vi "powermeter-main.vi"(3 "Perform Powermeter Auto Zero?":bool, 4 "error in (no error)":errorcluster, 5 "input-wavelength":i32, 6 "Set Wavelength?":bool, 7 "VISA in":refnum<visa-resource-name>="COM1") -> (0 "error out":errorcluster, 1 "output-wavelength":i32, 2 "power (µW)":dbl)   [LabVIEW 2015]
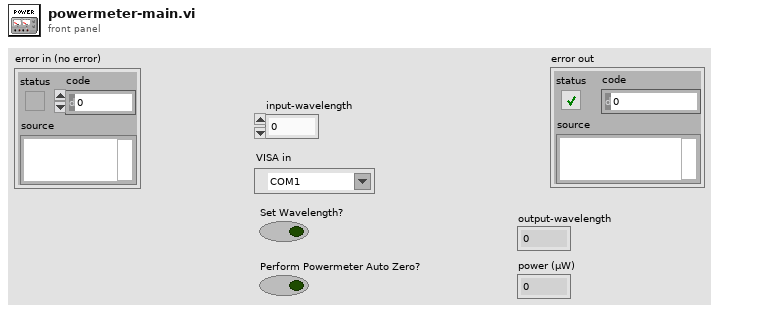
[diagram p1: front panel]
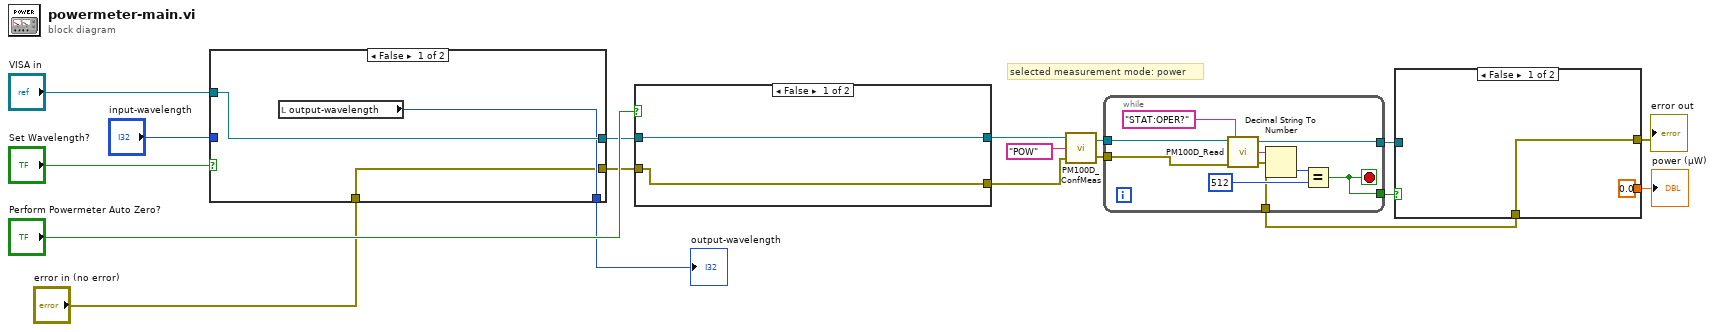
[diagram p0: block diagram]
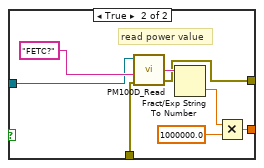
[diagram p2: hidden frame]
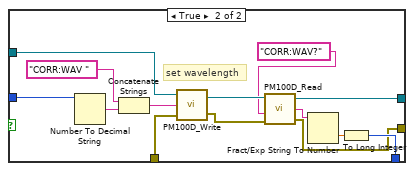
[diagram p3: hidden frame]
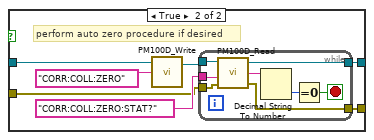
[diagram p4: hidden frame]
diagram:
  # "selected measurement mode: power"
  n1 = case shown="False" "Set Wavelength?" {
    tunnel: [w21 w29] -> w15
    tunnel: "VISA in" -> [w21 w32]
    tunnel: "input-wavelength" -> [_ w31]
    tunnel: [w20 w26] -> w9
    tunnel: "error in (no error)" -> [w19 w24]
    tunnel: [w19 w22] -> w5
    frame False {
      n2 = local read "output-wavelength"() -> (w20:i32)
    }
    frame True {
      # "set wavelength"
      n3 = Number To Decimal String(number=w31) -> (decimal integer string=w34:string)  [unwired: 1 in]
      n4 = Concatenate Strings("CORR:WAV " ("string"), w34) -> (w33:string)
      n5 = call "PM100D_Write.vi"("error in (no error)"=w24, "Command"=w33, "VISA in"=w32) -> ("error out"=w23:errorcluster, "VISA out"=w30:refnum<visa-resource-name>)
      n6 = call "PM100D_Read.vi"("error in (no error)"=w23, "Command"="CORR:WAV?" ("string"), "VISA in"=w30) -> ("error out"=w22:errorcluster, "ReadValue"=w27:string, "VISA out"=w29:refnum<visa-resource-name>)  [unwired: 1 in]
      n7 = Fract/Exp String To Number(string=w27) -> (number=w25:dbl)  [unwired: 3 in, 1 out]
      n8 = To Long Integer(number=w25) -> (32bit integer=w26:i32)
    }
  }
  "output-wavelength" <- w9
  n9 = case shown="False" "Perform Powermeter Auto Zero?" {
    tunnel: w15 -> [w37 w41]
    tunnel: [w37 w40] -> w11
    tunnel: w5 -> [w36 w39]
    tunnel: [w36 w38] -> w4
    frame False {
    }
    frame True {
      # "perform auto zero procedure if desired"
      n10 = call "PM100D_Write.vi"("Command"="CORR:COLL:ZERO" ("string"), "VISA in"=w41) -> ("VISA out"=w43:refnum<visa-resource-name>)  [unwired: 1 in, 1 out]
      n11 = while {
        tunnel: "CORR:COLL:ZERO:STAT?" ("string") -> [w48]
        tunnel: w43 -> [w49]
        tunnel: [w47] -> w40
        tunnel: w39 -> [w46]
        tunnel: [w45] -> w38
        stop <- w51 stop-if-true
        n12 = call "PM100D_Read.vi"("error in (no error)"=w46, "Command"=w48, "VISA in"=w49) -> ("error out"=w45:errorcluster, "ReadValue"=w50:string, "VISA out"=w47:refnum<visa-resource-name>)  [unwired: 1 in]
        n13 = Decimal String To Number(string=w50) -> (number=w52:i32)  [unwired: 2 in, 1 out]
        n14 = Equal To 0?(x=w52) -> (x = 0?=w51:bool)
      }
    }
  }
  n15 = call "PM100D_ConfMeas.vi"("error in"=w4, "Conf:"="POW", "VISA In"=w11) -> ("error out"=w3:errorcluster, "dup VISA session"=w12:refnum<visa-resource-name>)
  n16 = while {
    tunnel: w12 -> [w56]
    tunnel: [w57] -> w10
    tunnel: [w55] -> w7
    tunnel: w3 -> [w54]
    tunnel: [w53] -> w2
    stop <- w55 stop-if-true
    n17 = call "PM100D_Read.vi"("error in (no error)"=w54, "Command"="STAT:OPER?", "VISA in"=w56) -> ("error out"=w53:errorcluster, "ReadValue"=w59:string, "VISA out"=w57:refnum<visa-resource-name>)  [unwired: 1 in]
    n18 = Decimal String To Number(string=w59) -> (number=w60:i32)  [unwired: 2 in, 1 out]
    n19 = Equal?(x=w60, y=512) -> (x = y?=w55:bool)
  }
  n20 = case shown="False" w7 {
    tunnel: w10 -> [_ w69]
    tunnel: [0.0 w66] -> w8
    tunnel: w2 -> [w62 w65]
    tunnel: [w62 w64] -> w1
    frame False {
    }
    frame True {
      # "read power value"
      n21 = call "PM100D_Read.vi"("error in (no error)"=w65, "Command"="FETC?", "VISA in"=w69) -> ("error out"=w64:errorcluster, "ReadValue"=w71:string)  [unwired: 1 in, 1 out]
      n22 = Fract/Exp String To Number(string=w71) -> (number=w68:dbl)  [unwired: 3 in, 1 out]
      n23 = Multiply(x=w68, y=1000000.0) -> (x*y=w66:dbl)
    }
  }
  "power (µW)" <- w8
  "error out" <- w1
